vi "__updateWeather.vi"(10 "singleWeather":T1, 11 "BME280 in":refnum<class "BME280.lvclass">) -> (3 "BME280 out":refnum<class "BME280.lvclass">)   [LabVIEW 2020, in "BME280.lvclass"]
uses:
  BME280.lvclass
  Single Weather.ctl
  BME280.lvclass/BME280.ctl
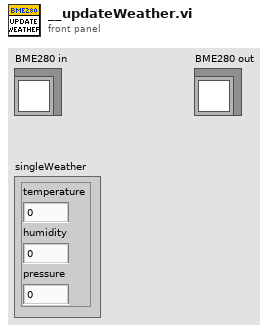
[diagram p1: front panel]
types:
  T1 = typedef "BME280.lvclass/Single Weather.ctl" = cluster{"temperature":dbl, "humidity":dbl, "pressure":dbl}
  T2 = typedef "BME280.lvclass/Weather.ctl" = cluster{"temperature":dbl[], "humidity":dbl[], "pressure":dbl[]}
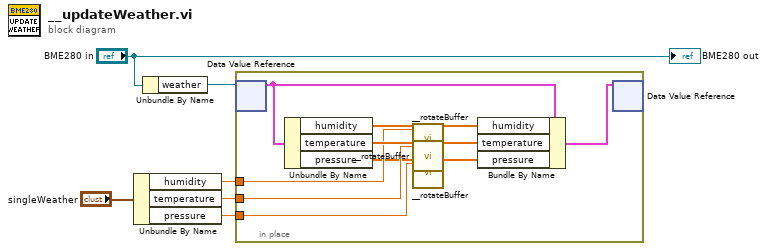
[diagram p0: block diagram]
diagram:
  n1 = Unbundle By Name("singleWeather") -> ("humidity"=w4:dbl, "temperature"=w3:dbl, "pressure"=w2:dbl)
  n2 = Unbundle By Name("BME280 in") -> ("weather"=w6:refnum<data-value>)
  n3 = in-place {
    in-place-border: w4 -> [w15]
    in-place-border: w3 -> [w14]
    in-place-border: w2 -> [w12]
    n4 = in-place-dvr #1(w6) -> (w11:T2)  [unwired: 1 out]
    n5 = Unbundle By Name(w11) -> ("humidity"=w16:dbl[], "temperature"=w17:dbl[], "pressure"=w13:dbl[])
    n6 = call "__rotateBuffer.vi"("data in"=w16, "new parameter"=w15) -> ("data out"=w10:dbl[])  [unwired: 25 in]
    n7 = call "__rotateBuffer.vi"("data in"=w17, "new parameter"=w14) -> ("data out"=w9:dbl[])  [unwired: 25 in]
    n8 = call "__rotateBuffer.vi"("data in"=w13, "new parameter"=w12) -> ("data out"=w8:dbl[])  [unwired: 25 in]
    n9 = Bundle By Name(cluster=w11, "humidity"=w10, "temperature"=w9, "pressure"=w8) -> (w7:T2)
    n10 = in-place-dvr #1(w7) -> ()  [unwired: 2 out]
  }
  "BME280 out" <- "BME280 in"
